vi "Ciclo while.vi"(0 "stop":bool) -> (1 "Indicatore numero":dbl, 2 "Iterazioni":dbl, 3 "Iterazioni (STOP)":dbl format="%#_3g", 4 "Tempo del\nciclo While":u32, 5 "Tempo tra inizio\ne pressione STOP":u32, 6 "Waveform Chart":dbl(graph))   [LabVIEW 2012]
panel:
  # "Realizzare un VI che rappresenta in un indicatore un valore casuale\n intero compreso  tra 0 e 100 in modo ripetuto.\n\nUna volta avviato, si deve poter terminare l'esecuzione del ciclo in \nqualunque istante, tramite un pulsante di stop.\n\nTale azione conclude il VI, visualizzando in uscita il numero delle \niterazioni effettuate."
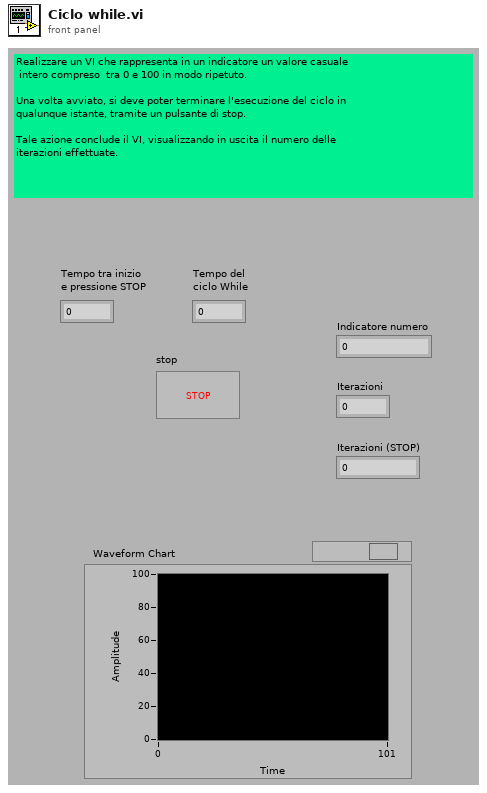
[diagram p1: front panel]
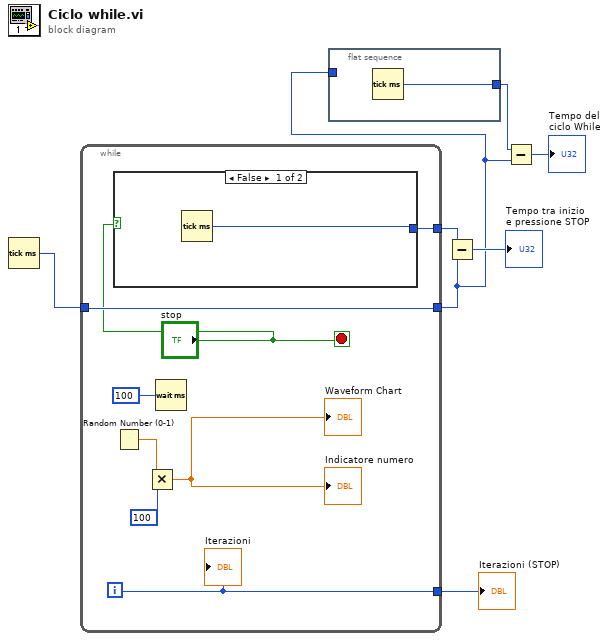
[diagram p0: block diagram]
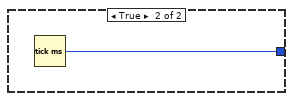
[diagram p2: hidden frame]
diagram:
  n1 = Tick Count (ms)() -> (millisecond timer value=w6:u32)
  n2 = while {
    tunnel: [w11] -> w7
    tunnel: w6 -> [w10]
    tunnel: [w10] -> w2
    tunnel: [w9] -> w4
    i -> [w11]
    stop <- "stop" stop-if-true
    n3 = case shown="False" "stop" {
      tunnel: [w16 w17] -> w9
      frame False {
        n4 = Tick Count (ms)() -> (millisecond timer value=w16:u32)
      }
      frame True {
        n5 = Tick Count (ms)() -> (millisecond timer value=w17:u32)
      }
    }
    n6 = Random Number (0-1)() -> (number: 0 to 1=w14:dbl)
    n7 = Multiply(x=w14, y=100) -> (x*y=→"Indicatore numero" →"Waveform Chart":dbl)
    n8 = Wait (ms)(milliseconds to wait=100) -> ()  [unwired: 1 out]
    "Iterazioni" <- w11
  }
  "Iterazioni (STOP)" <- w7
  n9 = flat-sequence {
    tunnel: w2 -> [_]
    tunnel: [w18] -> w3
    frame #0 {
      n10 = Tick Count (ms)() -> (millisecond timer value=w18:u32)
    }
  }
  n11 = Subtract(x=w4, y=w2) -> (x-y=→"Tempo tra inizio\ne pressione STOP":u32)
  n12 = Subtract(x=w3, y=w2) -> (x-y=→"Tempo del\nciclo While":u32)
